vi "Cartesian Increment Limits DAO.vi"(0 "Actions":T4, 3 "Config Ref Number":T3, 5 "LBCB Number":T1, 7 "Inc Limits In":T2, 11 "error in (no error)":errorcluster) -> (8 "Inc Limits Out":T2, 14 "Config Ref Number out":T3, 15 "error out":errorcluster)   [LabVIEW 2013]
uses:
  Metadata/Persistant DAO Actions.ctl
  Metadata/Cartesian Point.ctl
  <vilib>/Utility/config.llb/Config Data RefNum.ctl
  Metadata/LBCB Number.ctl
  <vilib>/Utility/config.llb/NI_LVConfig.lvlib
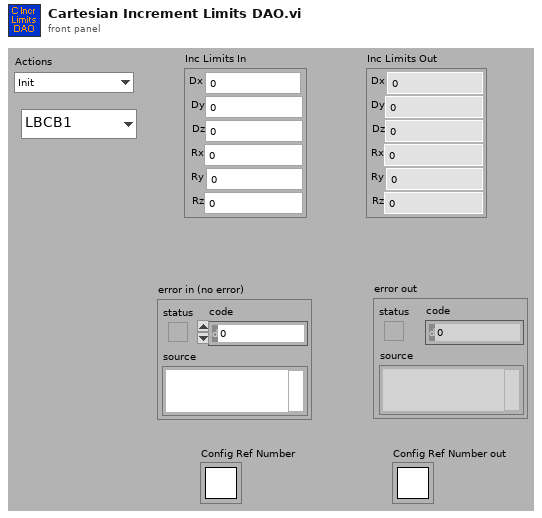
[diagram p1: front panel]
types:
  T1 = typedef "LBCB Number.ctl" = enum16{"LBCB1", "LBCB2"}
  T2 = typedef "Cartesian Point.ctl" = cluster{"Dx":dbl, "Dy":dbl, "Dz":dbl, "Rx":dbl, "Ry":dbl, "Rz":dbl}
  T3 = typedef "NI_LVConfig.lvlib/Config Data RefNum.ctl" = refnum<k1>
  T4 = typedef "Persistant DAO Actions.ctl" = enum16{"Init", "Get", "Set", "Load", "Save"}
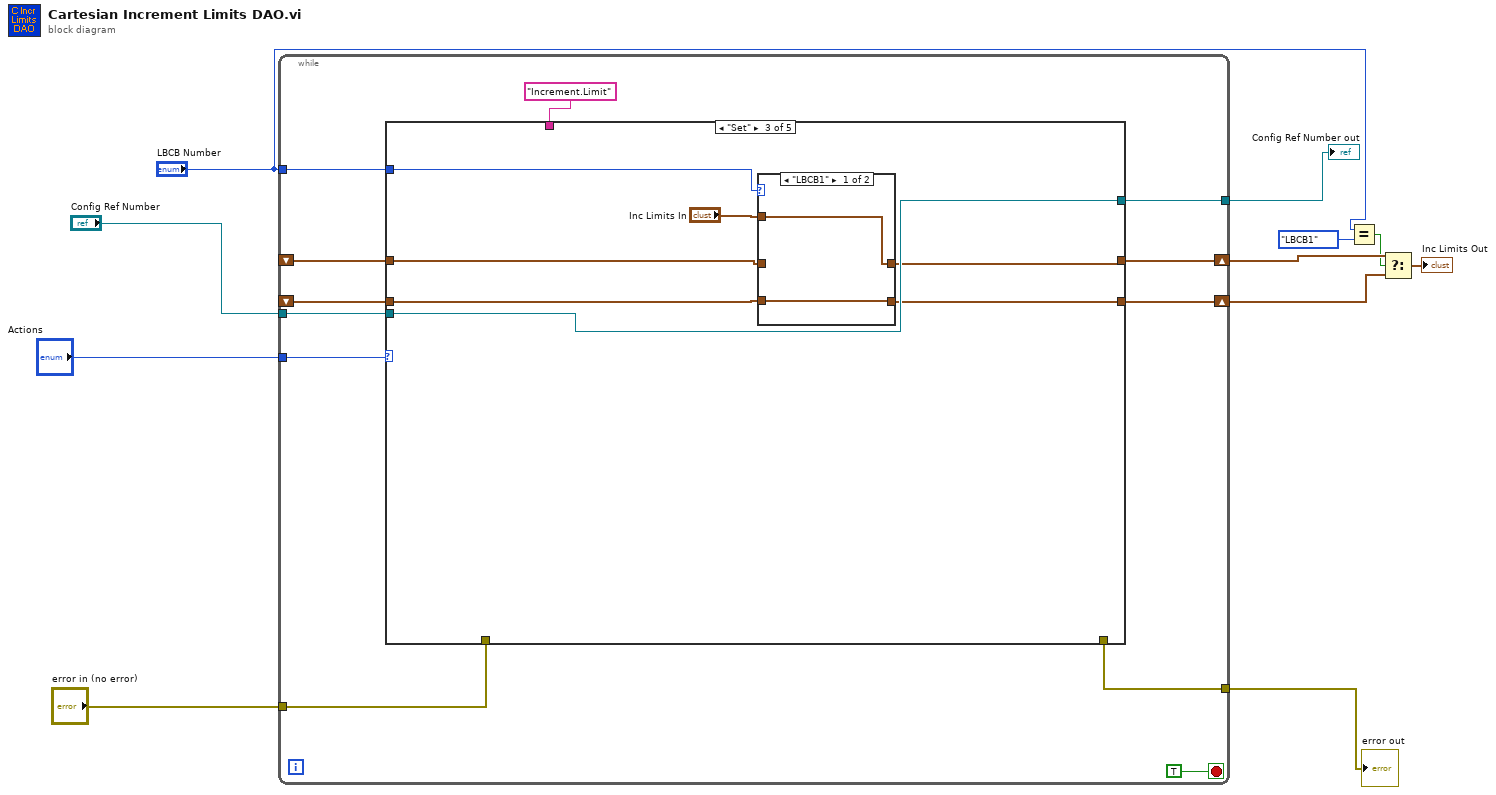
[diagram p0: block diagram]
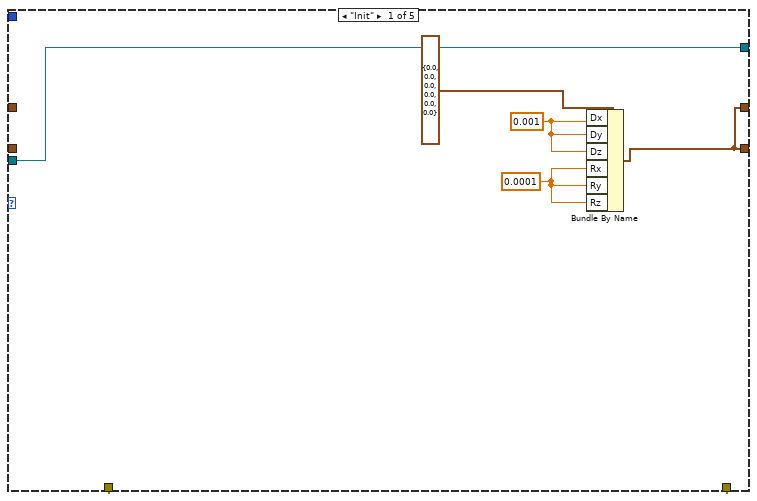
[diagram p2: hidden frame]
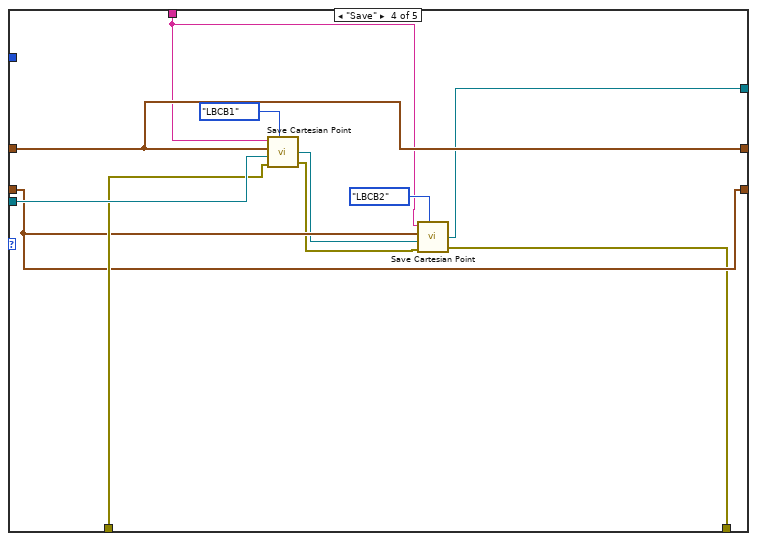
[diagram p5: hidden frame]
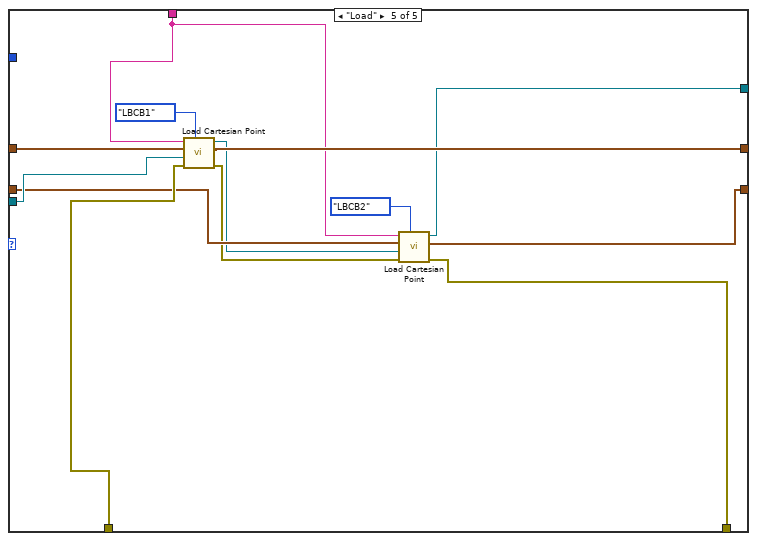
[diagram p6: hidden frame]
diagram:
  n1 = while {
    tunnel: "Actions" -> [w22]
    tunnel: "Config Ref Number" -> [w21]
    tunnel: "error in (no error)" -> [w19]
    tunnel: [w18] -> w8
    tunnel: [w17] -> w7
    shift-right: [w16] -> w5
    shift-left: _ -> [w15]
    tunnel: "LBCB Number" -> [w14]
    shift-right: [w13] -> w4
    shift-left: _ -> [w12]
    stop <- TRUE stop-if-true
    n2 = case shown="\"Set\"" w22 {
      tunnel: "Increment.Limit" ("section") -> [_ _ _ w51 w63]
      tunnel: w21 -> [w28 w32 w40 w56 w69]
      tunnel: w19 -> [w29 w33 w41 w55 w68]
      tunnel: [w28 w32 w40 w48 w60] -> w18
      tunnel: [w29 w33 w41 w46 w58] -> w17
      tunnel: [w26 w31 w34 w54 w66] -> w16
      tunnel: w15 -> [_ w31 w37 w54 w67]
      tunnel: w14 -> [_ _ w39 _ _]
      tunnel: [w26 w30 w35 w50 w57] -> w13
      tunnel: w12 -> [_ w30 w36 w50 w62]
      frame "Init" {
        w24 = 0.0001 ("X")
        w25 = 0.001 ("X")
        n3 = Bundle By Name(cluster=T2 {"Dx"=0.0, "Dy"=0.0, "Dz"=0.0, "Rx"=0.0, "Ry"=0.0, "Rz"=0.0} ("Max Increment Out"), "Dx"=w25, "Dy"=w25, "Dz"=w25, "Rx"=w24, "Ry"=w24, "Rz"=w24) -> (w26:T2)
      }
      frame "Get" {
      }
      frame "Set" {
        n4 = case shown="\"LBCB1\"" w39 {
          tunnel: "Inc Limits In" -> [w43 w45]
          tunnel: w37 -> [_ w44]
          tunnel: w36 -> [w42 _]
          tunnel: [w42 w45] -> w35
          tunnel: [w43 w44] -> w34
          frame "LBCB1" {
          }
          frame "LBCB2" {
          }
        }
      }
      frame "Save" {
        n5 = call "Save Cartesian Point.vi"("section"=w51, "Input Cluster"=w54, "refnum"=w56, "error in (no error)"=w55, "LBCB Number"=LBCB_Number."LBCB1") -> ("refnum out"=w49:T3, "error out"=w47:errorcluster)  [unwired: 1 out]
        n6 = call "Save Cartesian Point.vi"("section"=w51, "Input Cluster"=w50, "refnum"=w49, "error in (no error)"=w47, "LBCB Number"=LBCB_Number."LBCB2") -> ("refnum out"=w48:T3, "error out"=w46:errorcluster)  [unwired: 1 out]
      }
      frame "Load" {
        n7 = call "Load Cartesian Point.vi"("LBCB Number"=LBCB_Number."LBCB1", "error in (no error)"=w68, "refnum"=w69, "Input Cluster"=w67, "section"=w63) -> ("error out"=w59:errorcluster, "output cluster"=w66:T2, "refnum out"=w61:T3)  [unwired: 1 out]
        n8 = call "Load Cartesian Point.vi"("LBCB Number"=LBCB_Number."LBCB2", "error in (no error)"=w59, "refnum"=w61, "Input Cluster"=w62, "section"=w63) -> ("error out"=w58:errorcluster, "output cluster"=w57:T2, "refnum out"=w60:T3)  [unwired: 1 out]
      }
    }
  }
  "error out" <- w7
  "Config Ref Number out" <- w8
  n9 = Equal?(x="LBCB Number", y=LBCB_Number."LBCB1") -> (x = y?=w3:bool)
  n10 = Select(t=w5, s=w3, f=w4) -> (s? t:f=→"Inc Limits Out":T2)
